vi "TEST.vi"() -> ()   [LabVIEW 2016]
uses:
  <vilib>/vision/Image Controls.llb/IMAQ Image.ctl
  LV-EDSDK-Distribution_0.2/Distribution/EDSDK-Labview.llb/kEdsImageSrcs.ctl
  LV-EDSDK-Distribution_0.2/Distribution/EDSDK-Labview.llb/kEdsTargetImageTypes.ctl
  EDSDK131020CD(13.10.20)/EDSDK131020CD(13.10.20)/Windows/EDSDK_64/Dll/EDSDK.dll
  <vilib>/vision/NI_Vision_Development_Module.lvlib
panel:
  out "memoryStreamRef":u64
  out "dst":u8[](array[numeric])
  out "Array":u8[](array[numeric])
  out "Image out":T1
  out "appended array":u32[](array[numeric])
  out "2D Picture":picture
  out "Intensity Graph 2":i32[][](graph)
  in  "zoom":dbl
  out "Tv datatype":i32
  in  "Tv":u32
  out "Product Name":string
  out "PN datatype":i32
  out "destination":string
  out "initial":u32
  out "return type 9":u32
  out "return type 8":u32
  out "return type 7":u32
  out "return type 6":u32
  out "close session":u32
  out "get info/shutter button":u32
  out "open seeesion":u32
  out "get child":u32
  out "get list":u32
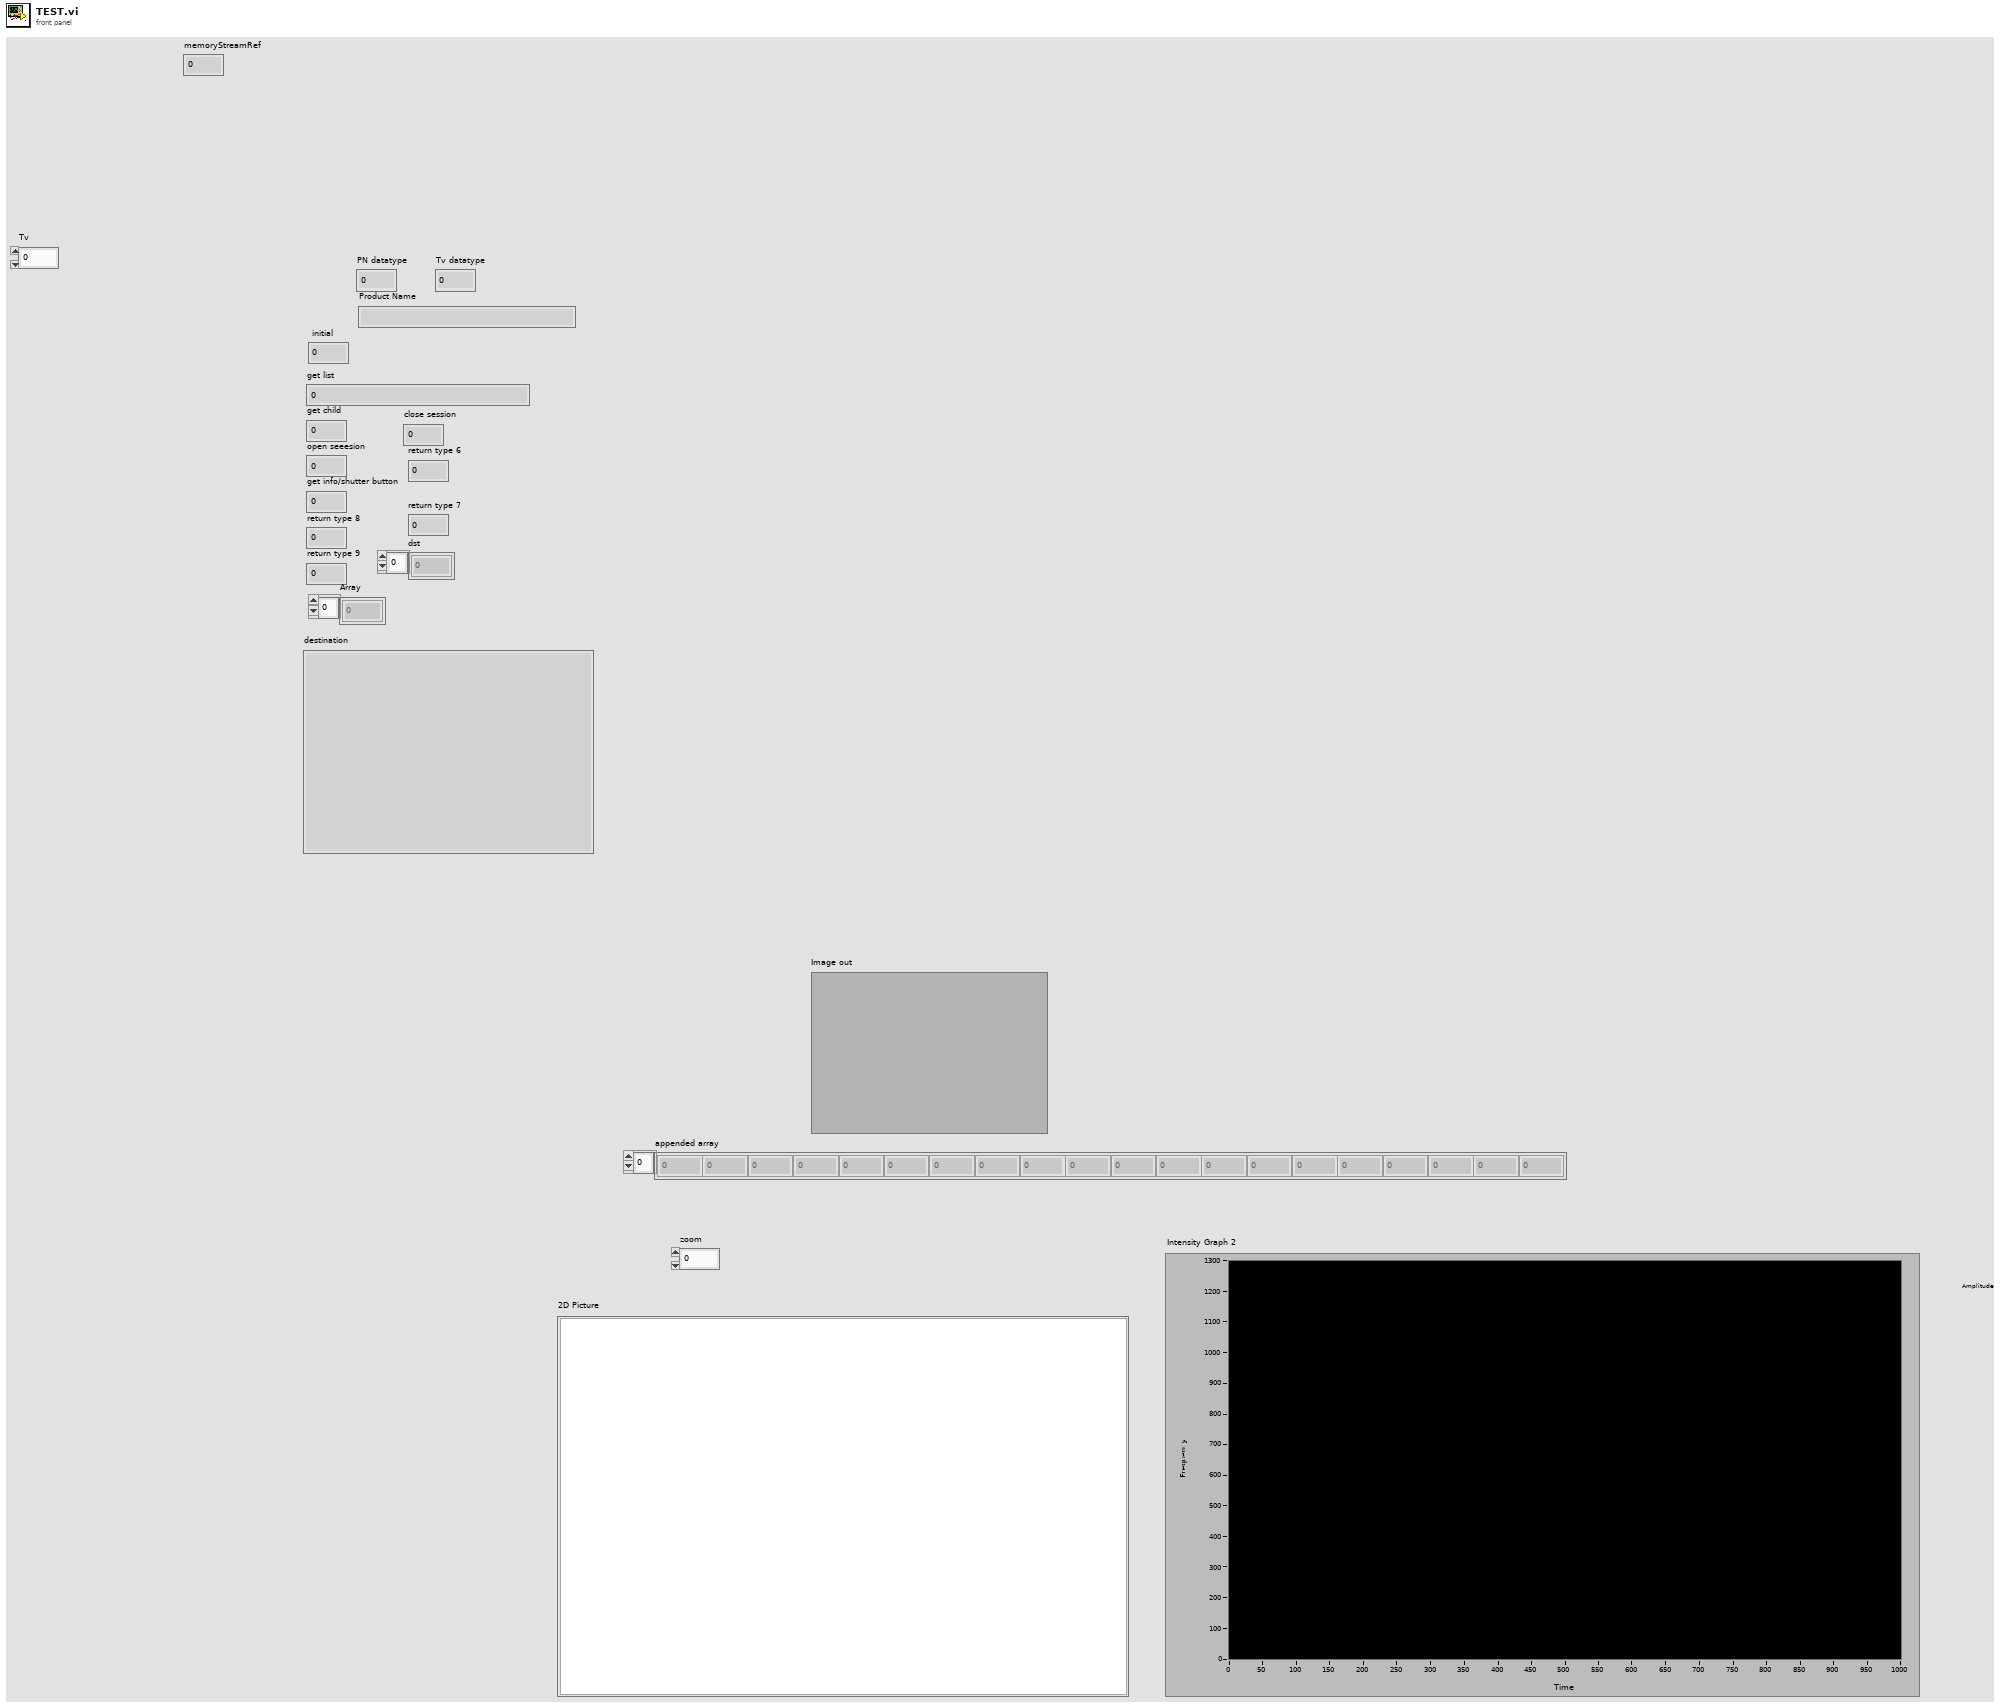
[diagram p1: front panel]
types:
  T1 = typedef "IMAQ Image.ctl" = refnum<image>
  T2 = cluster{cluster{"x":i32, "y":i32}, cluster{"width":i32, "height":i32}}
  T3 = cluster{"width":u32, "height":u32, "numofcompo":u32, "compoDepth":u32, cluster{cluster{"x":i32, "y":i32}, cluster{"width":i32, "height":i32}}, u32, u32}
  T4 = typedef "kEdsImageSrcs.ctl" = u32
  T5 = typedef "EdsImageInfo.ctl" = cluster{"width":u32, "height":u32, "# components":u32, "bit depth":u32, "rect":u32[], "reserved 1":u32, "reserved 2":u32}
  T6 = typedef "kEdsTargetImageTypes.ctl" = u32
  T7 = typedef "imagedata.ctl" = cluster{"image type":i32, "image depth":i32, "image":u8[], "mask":u8[], "colors":u32[], "Rectangle":cluster{"left":i16, "top":i16, "right":i16, "bottom":i16}}
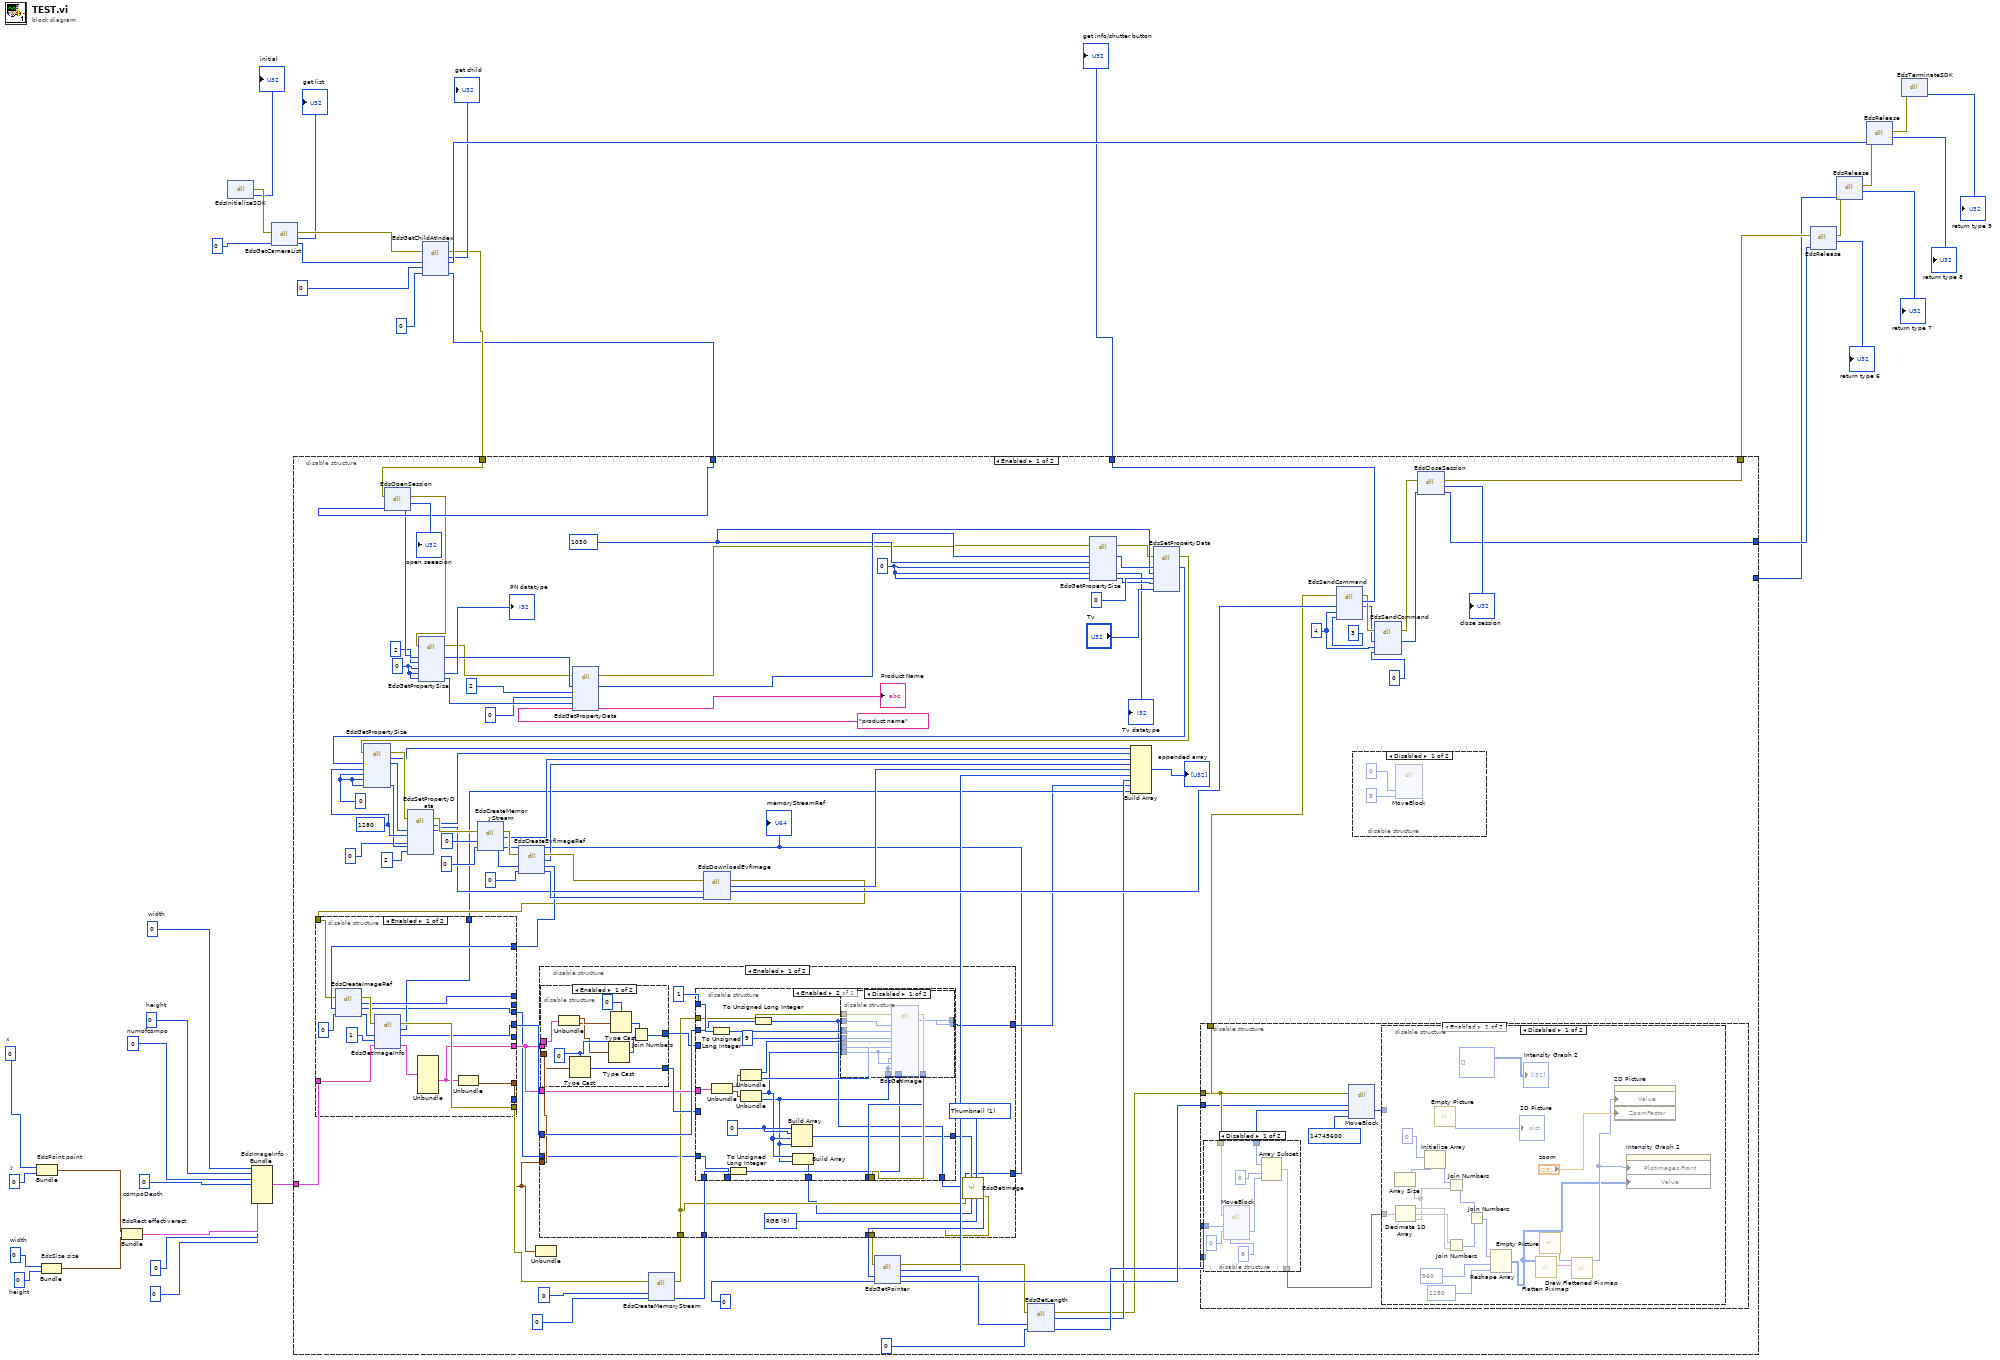
[diagram p0: block diagram]
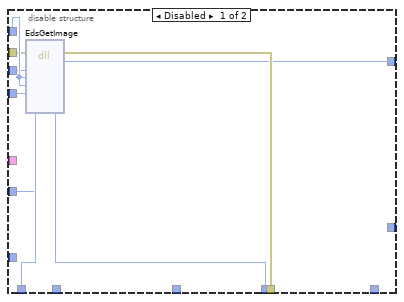
[diagram p2: hidden frame]
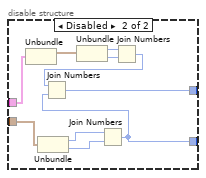
[diagram p4: hidden frame]
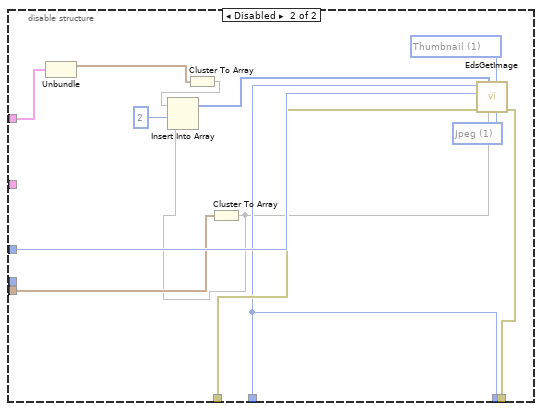
[diagram p5: hidden frame]
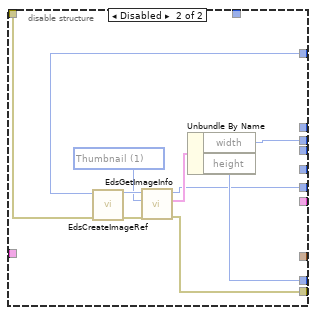
[diagram p7: hidden frame]
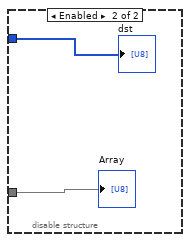
[diagram p9: hidden frame]
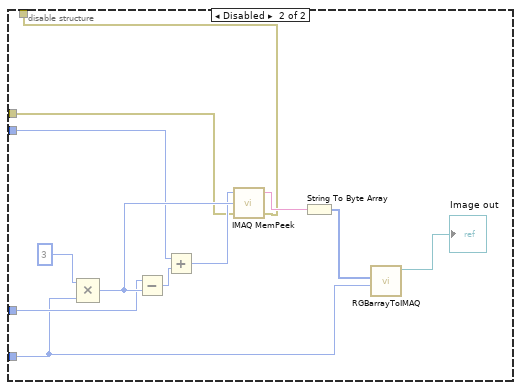
[diagram p10: hidden frame]
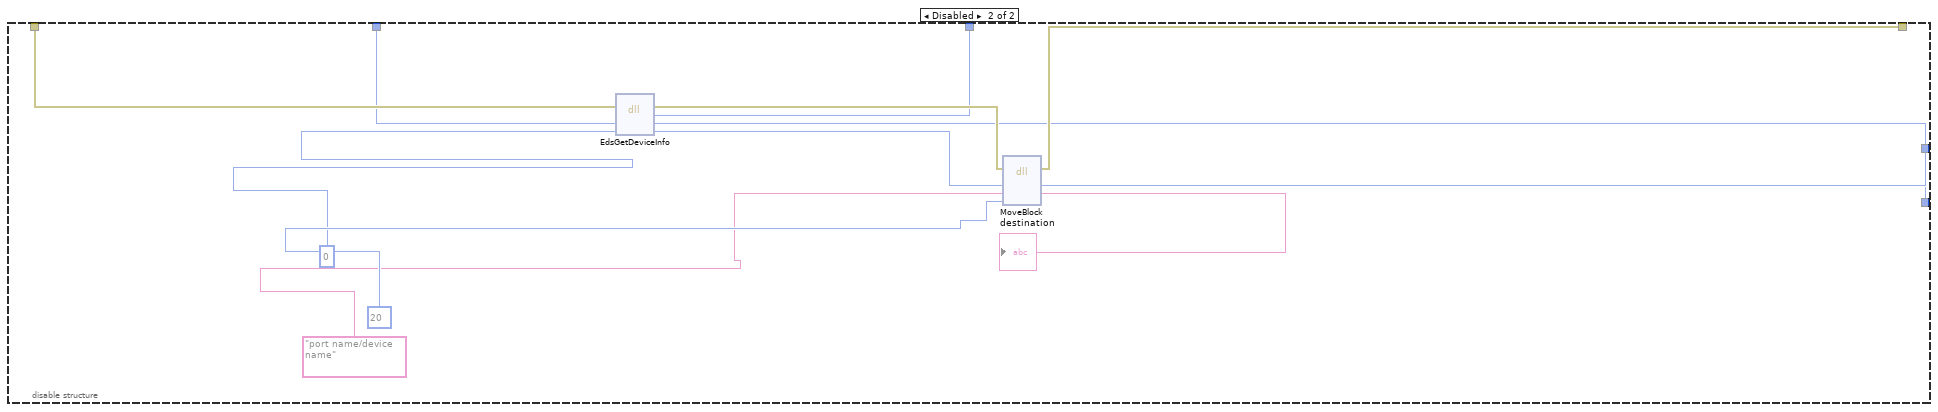
[diagram p11: hidden frame]
diagram:
  w11 = 0  # height
  w12 = 0  # width
  w13 = 0  # y
  w14 = 0  # x
  w7 = u32 0  # height
  w6 = u32 0  # numofcompo
  w5 = u32 0  # compoDepth
  w8 = u32 0  # width
  n1 = Bundle "EdsPoint point"("x"=w14, "y"=w13) -> (w10:cluster{"x":i32, "y":i32})  [unwired: 1 in]
  n2 = Bundle "EdsSize size"("width"=w12, "height"=w11) -> (w9:cluster{"width":i32, "height":i32})  [unwired: 1 in]
  n3 = Bundle "EdsRect effectiverect"(w10, w9) -> (w4:T2)  [unwired: 1 in]
  n4 = dll-call lib="D:/All Users/Summer2019/Camera_po_sheng/Canon/EDSDK131020CD(13.10.20)/EDSDK131020CD(13.10.20)/Windows/EDSDK_64/Dll/EDSDK.dll" fn="EdsInitializeSDK"() -> (error out=w37:errorcluster, "return type"=→"initial":u32)  [unwired: 3 in, 1 out]
  n5 = Bundle "EdsImageInfo"("width"=w8, "height"=w7, "numofcompo"=w6, "compoDepth"=w5, w4, u32 0, u32 0) -> (w1:T3)  [unwired: 1 in]
  n6 = dll-call lib="D:/All Users/Summer2019/Camera_po_sheng/Canon/EDSDK131020CD(13.10.20)/EDSDK131020CD(13.10.20)/Windows/EDSDK_64/Dll/EDSDK.dll" fn="EdsGetCameraList"(error in=w37, "CamListRef"=u64 0) -> (error out=w36:errorcluster, "return type"=→"get list":u32, "CamListRef"=w30:u64)  [unwired: 2 in, 1 out]
  n7 = dll-call lib="D:/All Users/Summer2019/Camera_po_sheng/Canon/EDSDK131020CD(13.10.20)/EDSDK131020CD(13.10.20)/Windows/EDSDK_64/Dll/EDSDK.dll" fn="EdsGetChildAtIndex"(error in=w36, "CamListRef"=w30, "index"=0, "CamRef"=u64 0) -> (error out=w20:errorcluster, "return type"=→"get child":u32, "CamListRef"=w32:u64, "CamRef"=w18:u64)  [unwired: 3 in, 1 out]
  n8 = disable-structure shown="Enabled" {
    disable-tunnel: w20 -> [w122 w302]
    disable-tunnel: [w121 w301] -> w19
    disable-tunnel: w18 -> [w120 w300]
    disable-tunnel: [w117 w299] -> w17
    disable-tunnel: [w119 w298] -> w16
    disable-tunnel: [_ w297] -> w15
    disable-tunnel: w1 -> [w52 _]
    frame Enabled {
      w84 = 0 ("para")
      w86 = u32 1280 ("PoropertyID")
      w98 = 0 ("para")
      w95 = u32 1030 ("PoropertyID")
      w108 = 0 ("para")
      w114 = u32 4 ("command")
      n9 = dll-call lib="D:/All Users/Summer2019/Camera_po_sheng/Canon/EDSDK131020CD(13.10.20)/EDSDK131020CD(13.10.20)/Windows/EDSDK_64/Dll/EDSDK.dll" fn="EdsOpenSession"(error in=w122, "CamRef"=w120) -> (error out=w106:errorcluster, "return type"=→"open seeesion":u32, "CamRef"=w110:u64)  [unwired: 2 in, 1 out]
      n10 = dll-call lib="D:/All Users/Summer2019/Camera_po_sheng/Canon/EDSDK131020CD(13.10.20)/EDSDK131020CD(13.10.20)/Windows/EDSDK_64/Dll/EDSDK.dll" fn="EdsGetPropertySize"(error in=w106, "CamRef"=w110, "PoropertyID"=u32 2, "para"=w108, "datatype"=w108, "size"=w108) -> (error out=w99:errorcluster, "CamRef"=w100:u64, "datatype"=→"PN datatype":i32, "size"=w103:u32)  [unwired: 5 in, 1 out]
      n11 = dll-call lib="D:/All Users/Summer2019/Camera_po_sheng/Canon/EDSDK131020CD(13.10.20)/EDSDK131020CD(13.10.20)/Windows/EDSDK_64/Dll/EDSDK.dll" fn="EdsGetPropertyData"(error in=w99, "CamRef"=w100, "PoropertyID"=u32 2, "para"=0, "size"=w103, "data"="product name") -> (error out=w89:errorcluster, "CamRef"=w96:u64, "data"=→"Product Name":string)  [unwired: 6 in, 1 out]
      n12 = dll-call lib="D:/All Users/Summer2019/Camera_po_sheng/Canon/EDSDK131020CD(13.10.20)/EDSDK131020CD(13.10.20)/Windows/EDSDK_64/Dll/EDSDK.dll" fn="EdsGetPropertySize"(error in=w89, "CamRef"=w96, "PoropertyID"=w95, "para"=w98, "datatype"=w98, "size"=w98) -> (error out=w90:errorcluster, "CamRef"=w97:u64, "datatype"=→"Tv datatype":i32, "size"=w93:u32)  [unwired: 5 in, 1 out]
      n13 = dll-call lib="D:/All Users/Summer2019/Camera_po_sheng/Canon/EDSDK131020CD(13.10.20)/EDSDK131020CD(13.10.20)/Windows/EDSDK_64/Dll/EDSDK.dll" fn="EdsSetPropertyData"(error in=w90, "CamRef"=w97, "PoropertyID"=w95, "para"=0, "size"=w93, "data"="Tv") -> (error out=w88:errorcluster, "CamRef"=w73:u64)  [unwired: 7 in, 1 out]
      n14 = dll-call lib="D:/All Users/Summer2019/Camera_po_sheng/Canon/EDSDK131020CD(13.10.20)/EDSDK131020CD(13.10.20)/Windows/EDSDK_64/Dll/EDSDK.dll" fn="EdsGetPropertySize"(error in=w88, "CamRef"=w73, "PoropertyID"=w86, "para"=w84, "datatype"=w84, "size"=w84) -> (error out=w87:errorcluster, "return type"=w66:u32, "CamRef"=w72:u64, "size"=w85:u32)  [unwired: 5 in, 1 out]
      n15 = dll-call lib="D:/All Users/Summer2019/Camera_po_sheng/Canon/EDSDK131020CD(13.10.20)/EDSDK131020CD(13.10.20)/Windows/EDSDK_64/Dll/EDSDK.dll" fn="EdsSetPropertyData"(error in=w87, "CamRef"=w72, "PoropertyID"=w86, "para"=0, "size"=w85, "data"=u32 2) -> (error out=w82:errorcluster, "return type"=w65:u32, "CamRef"=w75:u64)  [unwired: 6 in, 1 out]
      n16 = dll-call lib="D:/All Users/Summer2019/Camera_po_sheng/Canon/EDSDK131020CD(13.10.20)/EDSDK131020CD(13.10.20)/Windows/EDSDK_64/Dll/EDSDK.dll" fn="EdsCreateMemoryStream"(error in=w82, "size"=u64 0, "memoryStreamRef"=u64 0 ("StreamRef")) -> (error out=w79:errorcluster, "return type"=w64:u32, "memoryStreamRef"=w38:u64)  [unwired: 3 in, 1 out]
      "memoryStreamRef" <- w38
      n17 = dll-call lib="D:/All Users/Summer2019/Camera_po_sheng/Canon/EDSDK131020CD(13.10.20)/EDSDK131020CD(13.10.20)/Windows/EDSDK_64/Dll/EDSDK.dll" fn="EdsCreateEvfImageRef"(error in=w79, "memorystreamRef"=w38, "evfimageRef"=u64 0 ("evfstream")) -> (error out=w77:errorcluster, "return type"=w63:u32, "memorystreamRef"=w56:u64, "evfimageRef"=w76:u64)  [unwired: 2 in, 1 out]
      n18 = dll-call lib="D:/All Users/Summer2019/Camera_po_sheng/Canon/EDSDK131020CD(13.10.20)/EDSDK131020CD(13.10.20)/Windows/EDSDK_64/Dll/EDSDK.dll" fn="EdsDownloadEvfImage"(error in=w77, "CamRef"=w75, "evfimage"=w76) -> (error out=w54:errorcluster, "return type"=w62:u32, "CamRef"=w74:u64)  [unwired: 3 in, 1 out]
      n19 = disable-structure shown="Enabled" {
        disable-tunnel: w56 -> [w238 w244]
        disable-tunnel: [_ w243] -> _
        disable-tunnel: [_ w242] -> _
        disable-tunnel: [_ w241] -> _
        disable-tunnel: w54 -> [w234 w240]
        disable-tunnel: [w232 w239] -> w46
        disable-tunnel: [w231 _] -> _
        disable-tunnel: [w230 _] -> w53
        disable-tunnel: w52 -> [w229 _]
        disable-tunnel: [w228 _] -> w51
        disable-tunnel: [w226 _] -> w41
        disable-tunnel: [w225 _] -> w40
        disable-tunnel: [w224 _] -> w39
        frame Enabled {
          n20 = dll-call lib="D:/All Users/Summer2019/Camera_po_sheng/Canon/EDSDK131020CD(13.10.20)/EDSDK131020CD(13.10.20)/Windows/EDSDK_64/Dll/EDSDK.dll" fn="EdsCreateImageRef"(error in=w234, "streamRef"=w238, "imageRef"=u64 0) -> (error out=w233:errorcluster, "return type"=w231:u32, "streamRef"=w224:u64, "imageRef"=w236:u64)  [unwired: 2 in, 1 out]
          n21 = dll-call lib="D:/All Users/Summer2019/Camera_po_sheng/Canon/EDSDK131020CD(13.10.20)/EDSDK131020CD(13.10.20)/Windows/EDSDK_64/Dll/EDSDK.dll" fn="EdsGetImageInfo"(error in=w233, "imageRef"=w236, "imageSourse"=1, "InfoRef"=w229) -> (error out=w232:errorcluster, "return type"=w230:u32, "imageRef"=w228:u64, "InfoRef"=w227:T3)  [unwired: 3 in, 1 out]
          n22 = Unbundle(w227) -> (w225:T2)  [unwired: 6 out]
          n23 = Unbundle(w225) -> (w226:cluster{"width":i32, "height":i32})  [unwired: 1 out]
        }
        frame Disabled {
          w245 = T4 1 items=["FullView", "Thumbnail", "Preview", "RAWThumbnail", "RAWFullView"] ("inImageSource")
          n24 = call "EdsCreateImageRef.vi"("error in"=w240, "inStreamRef"=w244) -> ("error out"=w247:errorcluster, "outImageRef"=w246:u32)  [unwired: 8 in]
          n25 = call "EdsGetImageInfo.vi"("error in"=w247, "inImageSource"=w245, "inImageRef"=w246) -> ("error out"=w239:errorcluster, "outImageInfo"=w248:T5, "inImageRef dup"=w241:u32)  [unwired: 6 in]
          n26 = Unbundle By Name(w248) -> ("width"=w243:u32, "height"=w242:u32)
        }
      }
      n27 = Unbundle(w41) -> ()  [unwired: 2 out]
      n28 = dll-call lib="D:/All Users/Summer2019/Camera_po_sheng/Canon/EDSDK131020CD(13.10.20)/EDSDK131020CD(13.10.20)/Windows/EDSDK_64/Dll/EDSDK.dll" fn="EdsCreateMemoryStream"(error in=w46, "size"=u64 0, "memoryStreamRef"=u64 0 ("StreamRef")) -> (error out=w45:errorcluster, "memoryStreamRef"=w48:u64)  [unwired: 4 in, 1 out]
      n29 = disable-structure shown="Enabled" {
        disable-tunnel: w51 -> [w142 w219]
        disable-tunnel: w48 -> [w132 w216]
        disable-tunnel: [w135 w216] -> w47
        disable-tunnel: w45 -> [w131 w218]
        disable-tunnel: [w134 w217] -> w44
        disable-tunnel: [w141 _] -> w43
        disable-tunnel: w41 -> [w139 w213]
        disable-tunnel: w40 -> [w140 w212]
        disable-tunnel: w40 -> [w136 _]
        disable-tunnel: w39 -> [w126 _]
        disable-tunnel: w38 -> [w125 _]
        frame Enabled {
          w127 = T6 9 items=["Unknown"=0, "Jpeg"=1, "TIFF"=7, "TIFF16"=8, "RGB"=9, "RGB16"=10, "DIB"=11] ("inImageType")
          w129 = T4 1 items=["FullView", "Thumbnail", "Preview", "RAWThumbnail", "RAWFullView"] ("inImageSource")
          n30 = disable-structure shown="Enabled" {
            disable-tunnel: w140 -> [w193 w203]
            disable-tunnel: w139 -> [w196 w206]
            disable-tunnel: [w195 w198] -> w137
            disable-tunnel: [w187 w197] -> w138
            frame Enabled {
              w192 = u64 0
              n31 = Unbundle(w193) -> (w191:cluster{"x":i32, "y":i32}, w190:cluster{"width":i32, "height":i32})
              n32 = Type Cast(type=w192, x=w196) -> (*(type *) &x=w195:u64)
              n33 = Type Cast(type=w192, x=w190) -> (*(type *) &x=w188:u64)
              n34 = Type Cast(type=u64 0, x=w191) -> (*(type *) &x=w189:u64)
              n35 = Join Numbers(hi=w189, lo=w188) -> ((hi.lo)=w187:u64)
            }
            frame Disabled {
              n36 = Unbundle(w203) -> (w202:cluster{"x":i32, "y":i32})  [unwired: 1 out]
              n37 = Unbundle(w206) -> ("width"=w205:i32, "height"=w204:i32)
              n38 = Unbundle(w202) -> ("x"=w200:i32, "y"=w201:i32)
              n39 = Join Numbers(hi=w205, lo=w204) -> ((hi.lo)=w198:u64)
              n40 = Join Numbers(hi=w200, lo=w201) -> ((hi.lo)=w199:u64)
              n41 = Join Numbers(hi=w199, lo=w198) -> ((hi.lo)=w197:u64)
            }
          }
          n42 = disable-structure shown="Enabled" {
            disable-tunnel: 1 ("imagetype") -> [w152 w174]
            disable-tunnel: w142 -> [w151 w173]
            disable-tunnel: w132 -> [w150 w167]
            disable-tunnel: [w149 w163] -> _
            disable-tunnel: w131 -> [w148 w166]
            disable-tunnel: [w147 w165] -> _
            disable-tunnel: [w146 w164] -> w141
            disable-tunnel: w138 -> [w145 _]
            disable-tunnel: w137 -> [w144 _]
            disable-tunnel: w136 -> [_ w172]
            disable-tunnel: [_ w159] -> w133
            disable-tunnel: [_ w157] -> w130
            disable-tunnel: [_ w154] -> w128
            disable-tunnel: w126 -> [_ w153]
            disable-tunnel: [_ w153] -> _
            frame Disabled {
              n43 = dll-call lib="D:/All Users/Summer2019/Camera_po_sheng/Canon/EDSDK131020CD(13.10.20)/EDSDK131020CD(13.10.20)/Windows/EDSDK_64/Dll/EDSDK.dll" fn="EdsGetImage"(error in=w148, "imageRef"=w151, "imageSourse"=w152, "imagetype"=w152, "rect"=w145, "size"=w144, "outstream"=w150) -> (error out=w147:errorcluster, "return type"=w146:u32, "outstream"=w149:u64)  [unwired: 7 in, 1 out]
            }
            frame Enabled {
              w158 = 0 ("element")
              n44 = To Unsigned Long Integer(number=w174) -> (unsigned 32bit integer=w162:u32)
              n45 = Unbundle(w172) -> (w171:cluster{"x":i32, "y":i32}, w170:cluster{"width":i32, "height":i32})
              n46 = To Unsigned Long Integer(number=w167) -> (unsigned 32bit integer=w161:u32)
              n47 = Unbundle(w171) -> ("x"=w169:i32, "y"=w168:i32)
              n48 = Unbundle(w170) -> ("width"=w156:i32, "height"=w155:i32)
              n49 = To Unsigned Long Integer(number=w173) -> (unsigned 32bit integer=w159:u32)
              n50 = Build Array(w158, w158, w156, w155) -> (w157:i32[])
              n51 = Build Array(w156, w155) -> (w154:i32[])
              n52 = disable-structure shown="Disabled" {
                disable-tunnel: w169 -> [w186 _]
                disable-tunnel: w168 -> [w185 _]
                disable-tunnel: w156 -> [w184 _]
                disable-tunnel: w155 -> [w183 _]
                disable-tunnel: w166 -> [w182 _]
                disable-tunnel: [w181 _] -> w165
                disable-tunnel: [w180 _] -> w164
                disable-tunnel: [w179 _] -> w163
                disable-tunnel: w162 -> [w178 _]
                disable-tunnel: w161 -> [w177 _]
                disable-tunnel: u32 9 ("inImageType") -> [w176 _]
                disable-tunnel: w159 -> [w175 _]
                frame Disabled {
                  n53 = dll-call lib="D:/All Users/Summer2019/Camera_po_sheng/Canon/EDSDK131020CD(13.10.20)/EDSDK131020CD(13.10.20)/Windows/EDSDK_64/Dll/EDSDK.dll" fn="EdsGetImage"(error in=w182, "inImageRef"=w175, "inImageSource"=w178, "inImageType"=w176, "inSrcRect_x"=w186, "inSrcRect_y"=w185, "inSrcRect_sx"=w184, "inSrcRect_sy"=w183, "inDstSize_sx"=w184, "inDstSize_sy"=w183, "outStreamRef"=w177) -> (error out=w181:errorcluster, "return type"=w180:u32, "outStreamRef"=w179:u32)  [unwired: 11 in, 1 out]
                }
                frame Enabled {
                }
              }
            }
          }
          n54 = call "EdsGetImage.vi"("inImageType"=w127, "inImageSource"=w129, "inDstSize"=w128, "inSrcRect"=w130, "error in"=w131, "inImageRef"=w133, "inStreamRef"=w125) -> ("error out"=w134:errorcluster, "inStreamRef dup"=w135:u32)  [unwired: 3 in]
        }
        frame Disabled {
          w214 = T6 1 items=["Unknown"=0, "Jpeg"=1, "TIFF"=7, "TIFF16"=8, "RGB"=9, "RGB16"=10, "DIB"=11] ("inImageType")
          w215 = T4 1 items=["FullView", "Thumbnail", "Preview", "RAWThumbnail", "RAWFullView"] ("inImageSource")
          n55 = Unbundle(w212) -> (w211:cluster{"x":i32, "y":i32})  [unwired: 1 out]
          n56 = Cluster To Array(cluster=w211) -> (array=w210:i32[])
          n57 = Cluster To Array(cluster=w213) -> (array=w209:i32[])
          n58 = Insert Into Array(array=w210, index=2, new element=w209) -> (w208:i32[])
          n59 = call "EdsGetImage.vi"("inImageType"=w214, "inImageSource"=w215, "inDstSize"=w209, "inSrcRect"=w208, "error in"=w218, "inImageRef"=w219, "inStreamRef"=w216) -> ("error out"=w217:errorcluster)  [unwired: 3 in, 1 out]
        }
      }
      n60 = dll-call lib="D:/All Users/Summer2019/Camera_po_sheng/Canon/EDSDK131020CD(13.10.20)/EDSDK131020CD(13.10.20)/Windows/EDSDK_64/Dll/EDSDK.dll" fn="EdsGetPointer"(error in=w44, "streamRef"=w47, "pointer"=u64 0) -> (error out=w58:errorcluster, "return type"=w61:u32, "streamRef"=w55:u64, "pointer"=w71:u64)  [unwired: 2 in, 1 out]
      n61 = dll-call lib="D:/All Users/Summer2019/Camera_po_sheng/Canon/EDSDK131020CD(13.10.20)/EDSDK131020CD(13.10.20)/Windows/EDSDK_64/Dll/EDSDK.dll" fn="EdsGetLength"(error in=w58, "streamRef"=w55, "length"=u64 0 ("pointer")) -> (error out=w42:errorcluster, "return type"=w60:u32, "length"=w68:u64)  [unwired: 3 in, 1 out]
      n62 = Build Array(w66, w65, w64, w63, w62, w61, w60, w43, w53) -> (→"appended array":u32[])
      n63 = disable-structure shown="Enabled" {
        disable-tunnel: w71 -> [w249 w292]
        disable-tunnel: [w254 w285] -> w69
        disable-tunnel: w68 -> [w253 w293]
        disable-tunnel: _ -> [_ w288]
        disable-tunnel: w42 -> [w251 w286]
        frame Enabled {
          n64 = dll-call lib="LabVIEW" fn="MoveBlock"(error in=w251, "ptr"=w249, "size"=u64 14745600) -> (error out=w254:errorcluster, "dst"=w250:u8[])  [unwired: 6 in, 1 out]
          n65 = disable-structure shown="Disabled" {
            disable-tunnel: [w263 _] -> w255
            disable-tunnel: w253 -> [w262 _]
            disable-tunnel: w251 -> [w257 _]
            disable-tunnel: w250 -> [w256 _]
            frame Disabled {
              n66 = dll-call lib="LabVIEW" fn="MoveBlock"(error in=w257, "lenghPtr"=w262, "dst"=u64 0, "size"=u32 8) -> ("dst"=w258:u64)  [unwired: 5 in, 2 out]
              n67 = Array Subset(array=w256, index=0 ("y"), length=w258) -> (w263:u8[])
            }
            frame Enabled {
            }
          }
          n68 = disable-structure shown="Disabled" {
            disable-tunnel: w255 -> [w270 w284]
            disable-tunnel: w250 -> [_ w283]
            frame Disabled {
              n69 = Decimate 1D Array(w270) -> (w277:u8[], w278:u8[], w274:u8[])
              n70 = Array Size(array=w274) -> (size(s)=w273:i32)
              n71 = Initialize Array(u8 0 ("element"), w273) -> (w271:u8[])
              n72 = call "Empty Picture"() -> ("empty picture"=→"2D Picture":picture)
              n73 = Join Numbers(hi=w271, lo=w274) -> ((hi.lo)=w280:u16[])
              n74 = Join Numbers(hi=w278, lo=w277) -> ((hi.lo)=w279:u16[])
              n75 = Join Numbers(hi=w280, lo=w279) -> ((hi.lo)=w276:u32[])
              n76 = Reshape Array(w276, 960 ("dimension size"), 1280 ("dimension size")) -> (w265:u32[][])
              n77 = call <vilib>:"Flatten Pixmap.vi"("24-bit pixmap"=w265) -> ("image data"=w281:T7)  [unwired: 10 in]
              n78 = call "Empty Picture"() -> ("empty picture"=w282:picture)
              n79 = call <vilib>:"Draw Flattened Pixmap.vi"("image data"=w281, "picture"=w282) -> ("new picture"=w266:picture)  [unwired: 7 in]
              n80 = property on="2D Picture" class="Pict"("Value"=w266, "ZoomFactor"="zoom") -> ()  [unwired: 2 in, 2 out]
              n81 = property on="Intensity Graph 2" class="IntGraph (strict)"("PlotImages.Front"=w266, "Value"=w265) -> ()  [unwired: 2 in, 2 out]
              "Intensity Graph 2" <- i32[][] []
            }
            frame Enabled {
              "Array" <- w284
              "dst" <- w283
            }
          }
        }
        frame Disabled {
          n82 = Compound Arithmetic op=MULTIPLY(3 ("dimension size"), w288) -> (w294:u32)  [unwired: 1 in]
          n83 = Subtract(x=w293, y=w294) -> (x-y=w295:u64)
          n84 = Add(x=w292, y=w295) -> (x+y=w291:u64)
          n85 = call "IMAQ MemPeek"("error in (no error)"=w286, "Bytes count"=w294, "void*"=w291) -> ("error out"=w285:errorcluster, "Data string"=w290:string)  [unwired: 1 in]
          n86 = String To Byte Array(string=w290) -> (unsigned byte array=w289:u8[])
          n87 = call "RGBarrayToIMAQ.vi"("RGB vector (1D)"=w289, "height (for 1D)"=w288) -> ("Image out"=→"Image out":T1)  [unwired: 7 in]
        }
      }
      n88 = dll-call lib="D:/All Users/Summer2019/Camera_po_sheng/Canon/EDSDK131020CD(13.10.20)/EDSDK131020CD(13.10.20)/Windows/EDSDK_64/Dll/EDSDK.dll" fn="EdsSendCommand"(error in=w69, "camref"=w74, "command"=w114, "para"=u32 3) -> (error out=w116:errorcluster, "return type"=w117:u32, "camref"=w113:u64)  [unwired: 4 in, 1 out]
      n89 = disable-structure shown="Disabled" {
        frame Disabled {
          n90 = dll-call lib="LabVIEW" fn="MoveBlock"("dst"=u64 0, "size"=u32 8) -> ("Ptr"=w220:u64, "dst"=w223:u64)  [unwired: 6 in, 2 out]
        }
        frame Enabled {
        }
      }
      n91 = dll-call lib="D:/All Users/Summer2019/Camera_po_sheng/Canon/EDSDK131020CD(13.10.20)/EDSDK131020CD(13.10.20)/Windows/EDSDK_64/Dll/EDSDK.dll" fn="EdsSendCommand"(error in=w116, "camref"=w113, "command"=w114, "para"=u32 0) -> (error out=w115:errorcluster, "camref"=w111:u64)  [unwired: 5 in, 1 out]
      n92 = dll-call lib="D:/All Users/Summer2019/Camera_po_sheng/Canon/EDSDK131020CD(13.10.20)/EDSDK131020CD(13.10.20)/Windows/EDSDK_64/Dll/EDSDK.dll" fn="EdsCloseSession"(error in=w115, "CamRef"=w111) -> (error out=w121:errorcluster, "return type"=→"close session":u32, "CamRef"=w119:u64)  [unwired: 2 in, 1 out]
    }
    frame Disabled {
      n93 = dll-call lib="D:/All Users/Summer2019/Camera_po_sheng/Canon/EDSDK131020CD(13.10.20)/EDSDK131020CD(13.10.20)/Windows/EDSDK_64/Dll/EDSDK.dll" fn="EdsGetDeviceInfo"(error in=w302, "CamRef"=w300, "InfoRef"=u64 0) -> (error out=w308:errorcluster, "return type"=w299:u32, "CamRef"=w297:u64, "InfoRef"=w304:u64)  [unwired: 2 in, 1 out]
      n94 = dll-call lib="LabVIEW" fn="MoveBlock"(error in=w308, "pointer"=w304, "destination"="port name/device name", "size"=i64 20) -> (error out=w301:errorcluster, "pointer"=w298:i64, "destination"=→"destination":string)  [unwired: 4 in, 1 out]
    }
  }
  "get info/shutter button" <- w17
  n95 = dll-call lib="D:/All Users/Summer2019/Camera_po_sheng/Canon/EDSDK131020CD(13.10.20)/EDSDK131020CD(13.10.20)/Windows/EDSDK_64/Dll/EDSDK.dll" fn="EdsRelease"(error in=w19, "Ref"=w16) -> (error out=w34:errorcluster, "return type"=→"return type 6":u32)  [unwired: 3 in, 1 out]
  n96 = dll-call lib="D:/All Users/Summer2019/Camera_po_sheng/Canon/EDSDK131020CD(13.10.20)/EDSDK131020CD(13.10.20)/Windows/EDSDK_64/Dll/EDSDK.dll" fn="EdsRelease"(error in=w34, "Ref"=w15) -> (error out=w33:errorcluster, "return type"=→"return type 7":u32)  [unwired: 3 in, 1 out]
  n97 = dll-call lib="D:/All Users/Summer2019/Camera_po_sheng/Canon/EDSDK131020CD(13.10.20)/EDSDK131020CD(13.10.20)/Windows/EDSDK_64/Dll/EDSDK.dll" fn="EdsRelease"(error in=w33, "Ref"=w32) -> (error out=w31:errorcluster, "return type"=→"return type 8":u32)  [unwired: 3 in, 1 out]
  n98 = dll-call lib="D:/All Users/Summer2019/Camera_po_sheng/Canon/EDSDK131020CD(13.10.20)/EDSDK131020CD(13.10.20)/Windows/EDSDK_64/Dll/EDSDK.dll" fn="EdsTerminateSDK"(error in=w31) -> ("return type"=→"return type 9":u32)  [unwired: 2 in, 2 out]
